vi "Read Section - Path.vi"(4 "Default":path, 6 "Create file if not found? (T)":bool=TRUE, 7 "application directory":path, 8 "error in (no error)":errorcluster, 9 "key":string, 10 "section":string, 11 "Path":path) -> (0 "error out":errorcluster, 3 "value":path)   [LabVIEW 2019, in "TSC File IO.lvlib"]
doc: "This VI will read a section/cluster configuration file and return type path.\n\nThe VI will resolve relative paths that will be relative to the input ini file path and the symbolic path <appdir> which will use the input application directory or the application directory primative VI if blank. This gives flexibility to defining key/value pairs for absolute and relative paths.\n\nInputs:\n-Path [path] - a path to the file\n-section [string] - the section string in the configuration file\n-key [string] - the key to be read in the configuration file\n-error in\n\nOutputs:\n-value [path] - the output data read\n-error out\n_________________________________________________________________________\n<b>Code Developed By:</b>\nDaniel Coons\nTechnology Service Corporation\n1983 S Liberty Drive\nBloomington, IN 47403\nPhone: 812 558-7100\ndaniel.coons@tsc.com\nwww.tsc.com\n\n<b>Date Created:</b> 05 SEP 2014 \n<b>Date Updated:</b> 28 JUL 2021"
uses:
  TSC File IO.lvlib
  <vilib>/Utility/config.llb/NI_LVConfig.lvlib
  <vilib>/Utility/config.llb/Read Key (Path).vi
  <vilib>/Utility/sysdir.llb/System Directory Type.ctl
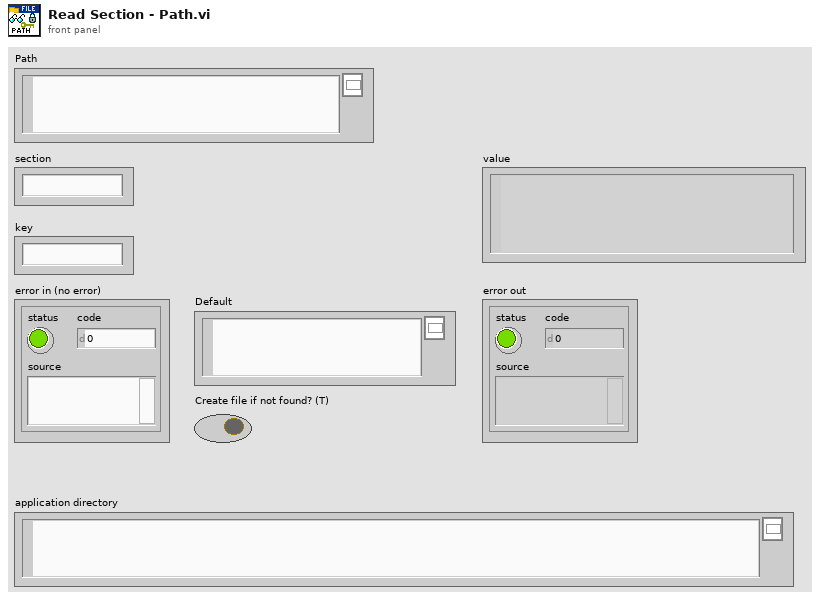
[diagram p1: front panel]
types:
  T1 = typedef "NI_LVConfig.lvlib/Config Data RefNum.ctl" = refnum<k1>
  T2 = typedef "System Directory Type.ctl" = i32
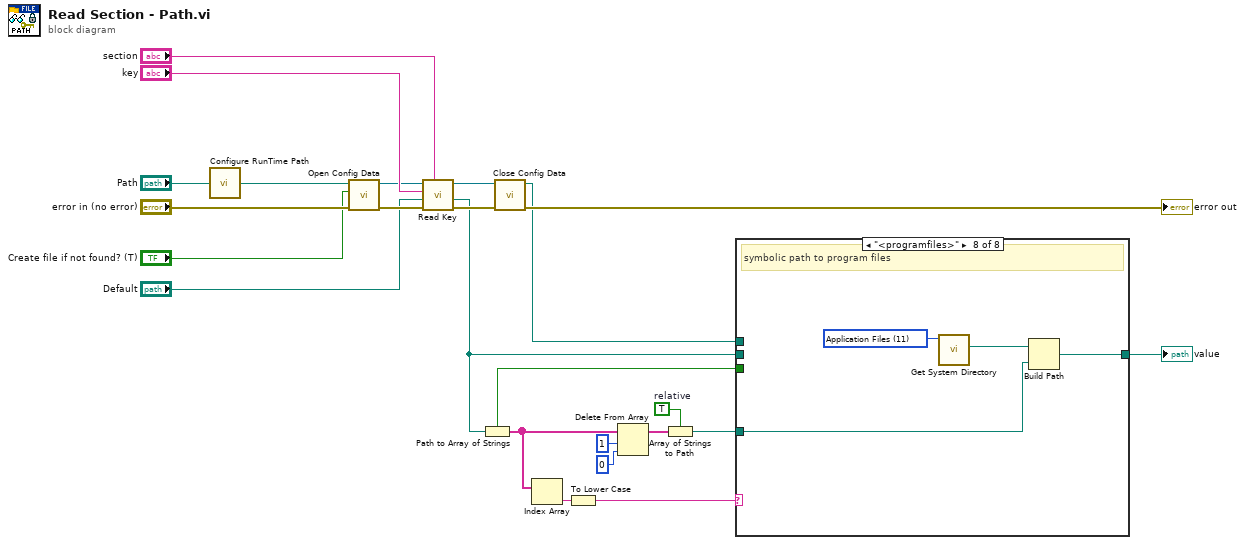
[diagram p0: block diagram]
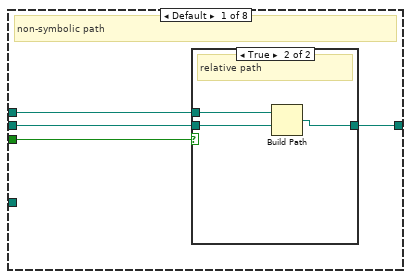
[diagram p2: hidden frame]
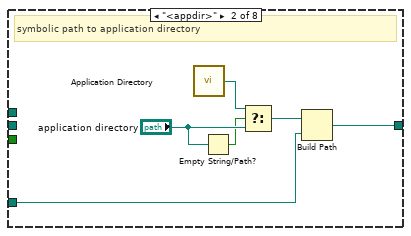
[diagram p4: hidden frame]
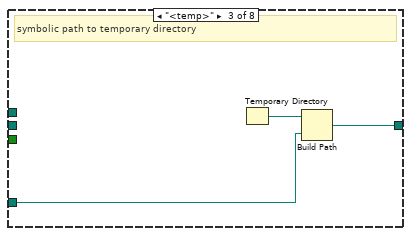
[diagram p5: hidden frame]
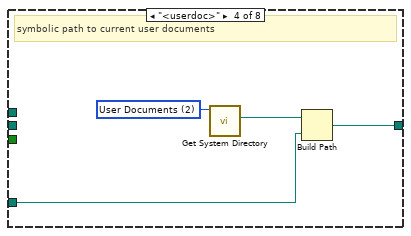
[diagram p6: hidden frame]
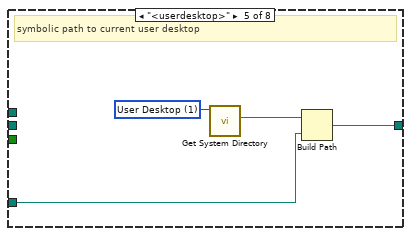
[diagram p7: hidden frame]
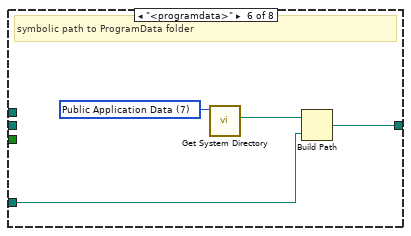
[diagram p8: hidden frame]
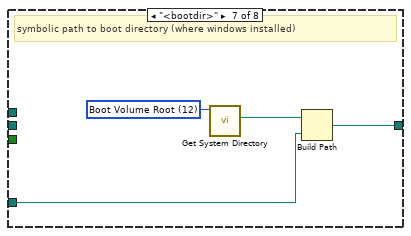
[diagram p9: hidden frame]
diagram:
  w5 = TRUE  # relative
  n1 = call "Configure RunTime Path.vi"("Input Path"="Path") -> ("Updated Path"=w16:path)
  n2 = call <vilib>:"Open Config Data.vi"("error in (no error)"="error in (no error)", "create file if necessary (T)"="Create file if not found? (T)", "configuration file path"=w16) -> ("error out"=w17:errorcluster, "refnum"=w18:T1)  [unwired: 6 in, 1 out]
  n3 = call-poly <vilib>:"Read Key.vi"("section"="section", "error in (no error)"=w17, "default value"="Default", "key"="key", "refnum"=w18) -> ("error out"=w19:errorcluster, "value"=w12:path, "refnum out"=w20:T1)  [unwired: 3 in, 1 out]
  n4 = Path to Array of Strings(0:w12) -> (1:w11:bool, 2:w1:string[])
  n5 = call <vilib>:"Close Config Data.vi"("error in (no error)"=w19, "refnum"=w20) -> ("error out"=→"error out":errorcluster, "file path"=w8:path)  [unwired: 8 in]
  n6 = Index Array(array=w1) -> (element=w13:string)  [unwired: 1 in]
  n7 = To Lower Case(string=w13) -> (all lower case string=w7:string)
  n8 = Delete From Array(array=w1, length=1, index=0) -> (array with subset deleted=w6:string[])  [unwired: 1 out]
  n9 = Array of Strings to Path(0:w6, 1:w5) -> (2:w2:path)
  n10 = case shown="\"<programfiles>\"" w7 {
    tunnel: w12 -> [w27 _ _ _ _ _ _ _]
    tunnel: w11 -> [w28 _ _ _ _ _ _ _]
    tunnel: [w26 w38 w41 w45 w49 w53 w57 w61] -> w10
    tunnel: w8 -> [w25 _ _ _ _ _ _ _]
    tunnel: w2 -> [_ w33 w39 w44 w48 w52 w56 w60]
    frame Default {
      # "non-symbolic path"
      n11 = case shown="True" w28 {
        tunnel: w27 -> [w29 w30]
        tunnel: [w29 w31] -> w26
        tunnel: w25 -> [_ w32]
        frame False {
          # "absolute path"
        }
        frame True {
          # "relative path"
          n12 = Build Path(base path=w32, name or relative path=w30) -> (appended path=w31:path)
        }
      }
    }
    frame "<appdir>" {
      # "symbolic path to application directory"
      n13 = call <vilib>:"Application Directory.vi"() -> ("Application Directory"=w37:path)
      n14 = Empty String/Path?(string/path="application directory") -> (empty?=w35:bool)
      n15 = Select(t=w37, s=w35, f="application directory") -> (s? t:f=w34:path)
      n16 = Build Path(base path=w34, name or relative path=w33) -> (appended path=w38:path)
    }
    frame "<temp>" {
      # "symbolic path to temporary directory"
      n17 = Temporary Directory() -> (w40:path)
      n18 = Build Path(base path=w40, name or relative path=w39) -> (appended path=w41:path)
    }
    frame "<userdoc>" {
      w43 = T2 2 items=["User Home"=0, "User Desktop"=1, "User Documents"=2, "User Application Data"=3, "User Preferences"=4, "User Temporary"=5, "Public Documents"=6, "Public Application Data"=7, "Public Preferences"=8, "Public Cache"=13, "System Core Libraries"=9, "System Installed Libraries"=10, "Application Files"=11, "Boot Volume Root"=12] ("system directory type")
      # "symbolic path to current user documents"
      n19 = call <vilib>:"Get System Directory.vi"("system directory type"=w43) -> ("system directory"=w42:path)  [unwired: 10 in]
      n20 = Build Path(base path=w42, name or relative path=w44) -> (appended path=w45:path)
    }
    frame "<userdesktop>" {
      w47 = T2 1 items=["User Home"=0, "User Desktop"=1, "User Documents"=2, "User Application Data"=3, "User Preferences"=4, "User Temporary"=5, "Public Documents"=6, "Public Application Data"=7, "Public Preferences"=8, "Public Cache"=13, "System Core Libraries"=9, "System Installed Libraries"=10, "Application Files"=11, "Boot Volume Root"=12] ("system directory type")
      # "symbolic path to current user desktop"
      n21 = call <vilib>:"Get System Directory.vi"("system directory type"=w47) -> ("system directory"=w46:path)  [unwired: 10 in]
      n22 = Build Path(base path=w46, name or relative path=w48) -> (appended path=w49:path)
    }
    frame "<programdata>" {
      w51 = T2 7 items=["User Home"=0, "User Desktop"=1, "User Documents"=2, "User Application Data"=3, "User Preferences"=4, "User Temporary"=5, "Public Documents"=6, "Public Application Data"=7, "Public Preferences"=8, "Public Cache"=13, "System Core Libraries"=9, "System Installed Libraries"=10, "Application Files"=11, "Boot Volume Root"=12] ("system directory type")
      # "symbolic path to ProgramData folder"
      n23 = call <vilib>:"Get System Directory.vi"("system directory type"=w51) -> ("system directory"=w50:path)  [unwired: 10 in]
      n24 = Build Path(base path=w50, name or relative path=w52) -> (appended path=w53:path)
    }
    frame "<bootdir>" {
      w55 = T2 12 items=["User Home"=0, "User Desktop"=1, "User Documents"=2, "User Application Data"=3, "User Preferences"=4, "User Temporary"=5, "Public Documents"=6, "Public Application Data"=7, "Public Preferences"=8, "Public Cache"=13, "System Core Libraries"=9, "System Installed Libraries"=10, "Application Files"=11, "Boot Volume Root"=12] ("system directory type")
      # "symbolic path to boot directory (where windows installed)"
      n25 = call <vilib>:"Get System Directory.vi"("system directory type"=w55) -> ("system directory"=w54:path)  [unwired: 10 in]
      n26 = Build Path(base path=w54, name or relative path=w56) -> (appended path=w57:path)
    }
    frame "<programfiles>" {
      w59 = T2 11 items=["User Home"=0, "User Desktop"=1, "User Documents"=2, "User Application Data"=3, "User Preferences"=4, "User Temporary"=5, "Public Documents"=6, "Public Application Data"=7, "Public Preferences"=8, "Public Cache"=13, "System Core Libraries"=9, "System Installed Libraries"=10, "Application Files"=11, "Boot Volume Root"=12] ("system directory type")
      # "symbolic path to program files"
      n27 = call <vilib>:"Get System Directory.vi"("system directory type"=w59) -> ("system directory"=w58:path)  [unwired: 10 in]
      n28 = Build Path(base path=w58, name or relative path=w60) -> (appended path=w61:path)
    }
  }
  "value" <- w10
